vi "Post-Build Action.vi"(5 "Files Generated by Build":path[](array[path]), 6 "Top Level/Always Included VIs":path[](array[path]), 7 "Destination Path":path, 8 "error in (no error)":errorcluster, 9 "Target Name":string, 10 "Build Specification Name":string, 11 "Project Path":path) -> (0 "error out":errorcluster)   [LabVIEW 2017]
uses:
  <vilib>/Utility/sysdir.llb/System Directory Type.ctl
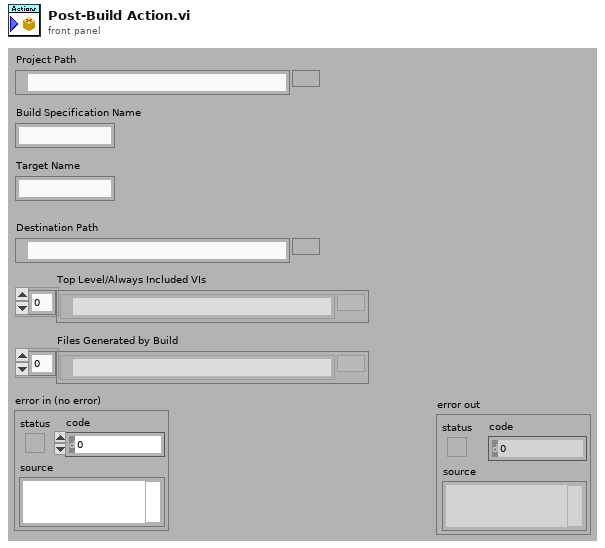
[diagram p1: front panel]
types:
  T1 = typedef "System Directory Type.ctl" = i32
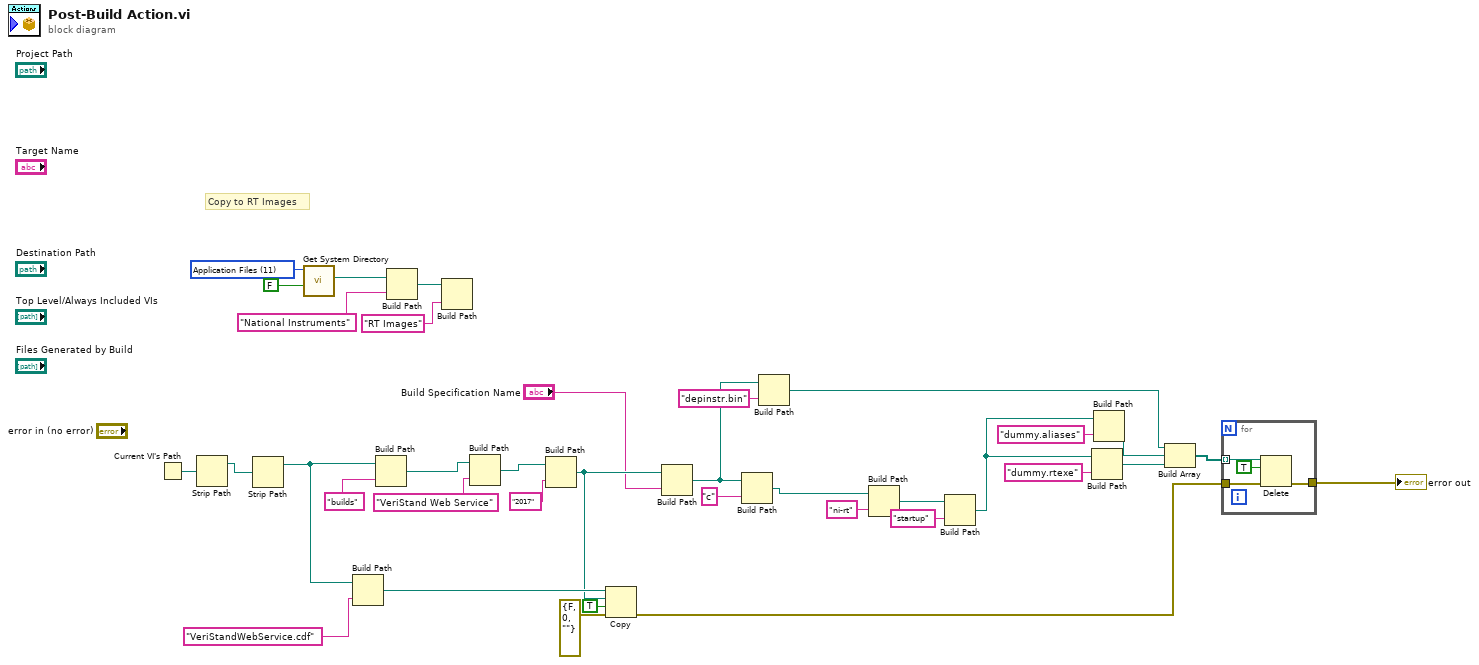
[diagram p0: block diagram]
diagram:
  w36 = T1 11 items=["User Home"=0, "User Desktop"=1, "User Documents"=2, "User Application Data"=3, "User Preferences"=4, "User Temporary"=5, "Public Documents"=6, "Public Application Data"=7, "Public Preferences"=8, "Public Cache"=13, "System Core Libraries"=9, "System Installed Libraries"=10, "Application Files"=11, "Boot Volume Root"=12] ("system directory type")
  # "Copy to RT Images"
  n1 = Current VI's Path() -> (path=w30:path)
  n2 = Strip Path(path=w30) -> (stripped path=w29:path)  [unwired: 1 out]
  n3 = Strip Path(path=w29) -> (stripped path=w16:path)  [unwired: 1 out]
  n4 = call <vilib>:"Get System Directory.vi"("create directory if not found? (F)"=FALSE, "system directory type"=w36) -> ("system directory"=w34:path)  [unwired: 9 in]
  n5 = Build Path(base path=w16, name or relative path="VeriStandWebService.cdf") -> (appended path=w10:path)
  n6 = Build Path(base path=w16, name or relative path="builds") -> (appended path=w15:path)
  n7 = Build Path(base path=w34, name or relative path="National Instruments") -> (appended path=w32:path)
  n8 = Build Path(base path=w32, name or relative path="RT Images") -> ()  [unwired: 1 out]
  n9 = Build Path(base path=w15, name or relative path="VeriStand Web Service") -> (appended path=w14:path)
  n10 = Build Path(base path=w14, name or relative path="2017") -> (appended path=w9:path)
  n11 = Copy(8:errorcluster {"status"=FALSE, "code"=0, "source"=""} ("error out"), 9:TRUE ("overwrite (F)"), 10:w9, 11:w10) -> (0:w7:errorcluster)  [unwired: 1 in, 2 out]
  n12 = Build Path(base path=w9, name or relative path="Build Specification Name") -> (appended path=w5:path)
  n13 = Build Path(base path=w5, name or relative path="c") -> (appended path=w11:path)
  n14 = Build Path(base path=w5, name or relative path="depinstr.bin") -> (appended path=w3:path)
  n15 = Build Path(base path=w11, name or relative path="ni-rt") -> (appended path=w24:path)
  n16 = Build Path(base path=w24, name or relative path="startup") -> (appended path=w20:path)
  n17 = Build Path(base path=w20, name or relative path="dummy.rtexe") -> (appended path=w18:path)
  n18 = Build Path(base path=w20, name or relative path="dummy.aliases") -> (appended path=w19:path)
  n19 = Build Array(w3, w19, w18) -> (w17:path[])
  n20 = for {
    tunnel: w17 -> [w40] mode=indexing
    tunnel: w7 -> [w39]
    tunnel: [w38] -> w6
    n21 = Delete(path (use dialog)=w40, entire hierarchy (F)=TRUE, error in=w39) -> (error out=w38:errorcluster)  [unwired: 2 in, 2 out]
  }
  "error out" <- w6
